vi "表格行数.vi"(3 "E检定表格":string[][](table)=[["", "", "", "", ""], ["", "", "", "", ""], ["", "", "", "", ""], ["", "", "", "", ""], ["", "", "", "", ""]]) -> (1 "行数":i32)   [LabVIEW 2014]
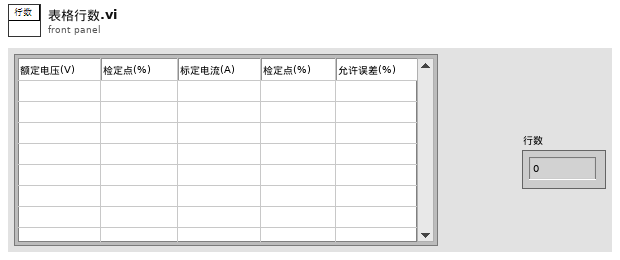
[diagram p1: front panel]
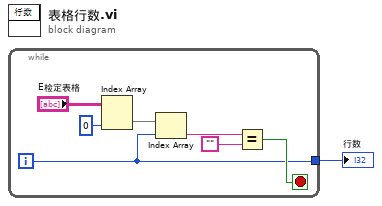
[diagram p0: block diagram]
diagram:
  n1 = while {
    tunnel: [w3] -> w1
    i -> [w3]
    stop <- w4 stop-if-true
    n2 = Index Array(array="E检定表格", index (col)=0 ("禁用的索引 (列)")) -> (element=w7:string[])  [unwired: 1 in]
    n3 = Index Array(array=w7, index=w3) -> (element=w6:string)
    n4 = Equal?(x=w6, y="") -> (x = y?=w4:bool)
  }
  "行数" <- w1
